vi "load_calib.vi"(11 "Calibrate Spectrum":path) -> (0 "Param Calib":T1, 1 "List":dbl[][](array[numeric]), 2 "Table":string[][](array[string]), 3 "Spectrum Out":cluster{"all rows":dbl[], "all rows":dbl[]}, 4 "List Parameter Fit Out":dbl[][](array[numeric]))   [LabVIEW 2023]
uses:
  control/param_calibrazione.ctl
  <vilib>/Utility/file.llb/Read Delimited Spreadsheet (DBL).vi
  <vilib>/Utility/file.llb/Read Delimited Spreadsheet (string).vi
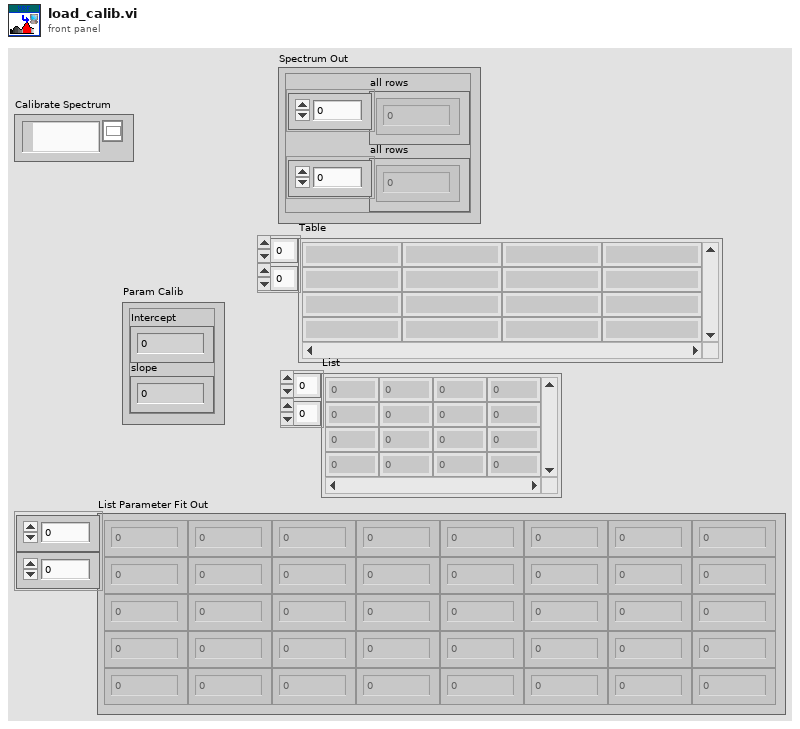
[diagram p1: front panel]
types:
  T1 = typedef "param_calibrazione.ctl" = cluster{"Intercept":dbl, "slope":dbl}
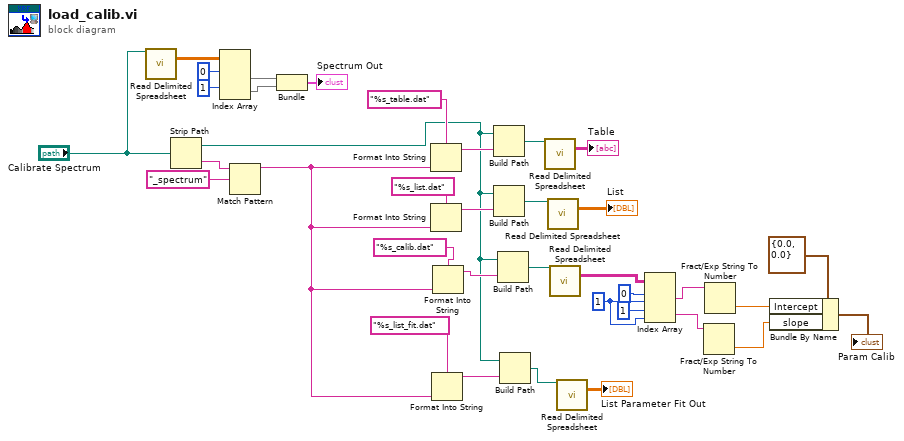
[diagram p0: block diagram]
diagram:
  w14 = 1 ("disabled index (col)")
  n1 = call-poly <vilib>:"Read Delimited Spreadsheet.vi"("file path (dialog if empty)"="Calibrate Spectrum") -> ("all rows"=w28:dbl[][])  [unwired: 9 in, 5 out]
  n2 = Strip Path(path="Calibrate Spectrum") -> (stripped path=w3:path, name=w32:string)
  n3 = Index Array(array=w28, index (row) #1=0 ("index (row)"), index (row) #2=1 ("index (row)")) -> (element #1=w24:dbl[], element #2=w25:dbl[])  [unwired: 2 in]
  n4 = Match Pattern(string=w32, regular expression="_spectrum") -> (before substring=w5:string)  [unwired: 1 in, 3 out]
  n5 = Bundle("all rows"=w24, "all rows"=w25) -> (→"Spectrum Out":cluster{"all rows":dbl[], "all rows":dbl[]})  [unwired: 1 in]
  n6 = Format Into String(format string="%s_table.dat", w5) -> (resulting string=w34:string)  [unwired: 2 in, 1 out]
  n7 = Format Into String(format string="%s_list.dat", w5) -> (resulting string=w33:string)  [unwired: 2 in, 1 out]
  n8 = Format Into String(format string="%s_list_fit.dat", w5) -> (resulting string=w4:string)  [unwired: 2 in, 1 out]
  n9 = Format Into String(format string="%s_calib.dat", w5) -> (resulting string=w18:string)  [unwired: 2 in, 1 out]
  n10 = Build Path(base path=w3, name or relative path=w34) -> (appended path=w36:path)
  n11 = Build Path(base path=w3, name or relative path=w33) -> (appended path=w35:path)
  n12 = Build Path(base path=w3, name or relative path=w18) -> (appended path=w17:path)
  n13 = Build Path(base path=w3, name or relative path=w4) -> (appended path=w2:path)
  n14 = call-poly <vilib>:"Read Delimited Spreadsheet.vi"("file path (dialog if empty)"=w36) -> ("all rows"=→"Table":string[][])  [unwired: 9 in, 5 out]
  n15 = call-poly <vilib>:"Read Delimited Spreadsheet.vi"("file path (dialog if empty)"=w35) -> ("all rows"=→"List":dbl[][])  [unwired: 9 in, 5 out]
  n16 = call-poly <vilib>:"Read Delimited Spreadsheet.vi"("file path (dialog if empty)"=w17) -> ("all rows"=w11:string[][])  [unwired: 9 in, 5 out]
  n17 = call-poly <vilib>:"Read Delimited Spreadsheet.vi"("file path (dialog if empty)"=w2) -> ("all rows"=→"List Parameter Fit Out":dbl[][])  [unwired: 9 in, 5 out]
  n18 = Index Array(array=w11, index (row) #1=0 ("index (row)"), index (col) #1=w14, index (row) #2=1 ("index (row)"), index (col) #2=w14) -> (element #1=w13:string, element #2=w12:string)
  n19 = Fract/Exp String To Number(string=w12) -> (number=w7:dbl)  [unwired: 3 in, 1 out]
  n20 = Fract/Exp String To Number(string=w13) -> (number=w8:dbl)  [unwired: 3 in, 1 out]
  n21 = Bundle By Name(cluster=T1 {"Intercept"=0.0, "slope"=0.0} ("param_calib"), "Intercept"=w8, "slope"=w7) -> (→"Param Calib":T1)
